vi "ad get drv version.vi"(8 "error in (no error)":errorcluster, 10 "vers":u32, 11 "adh":i32) -> (0 "error out":errorcluster, 2 "vers out":u32, 3 "function return":i32)   [LabVIEW 2021, in "libad4.lvlib"]
doc: "ad_get_drv_version (int32_t adh, uint32_t *vers);\n\nIndicates what version of the DAQ driver LIBAD4 is compatible with."
uses:
  <userlib>/libad4/libad4.lvlib
  <userlib>/libad4/libad4.dll
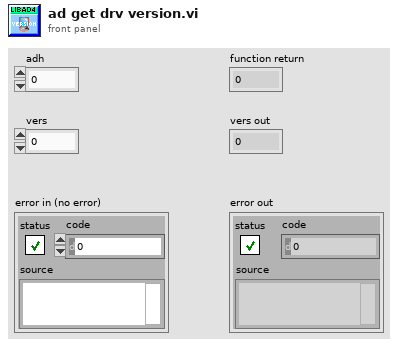
[diagram p1: front panel]
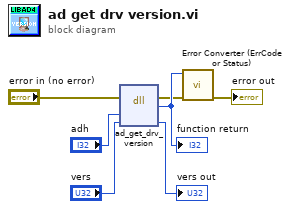
[diagram p0: block diagram]
diagram:
  n1 = dll-call lib="C:/Program Files/National Instruments/LabVIEW 2021/user.lib/libad4/libad4.*" fn="ad_get_drv_version"(error in="error in (no error)", "adh"="adh", "vers"="vers") -> (error out=w2:errorcluster, w7:i32, "vers"=→"vers out":u32)  [unwired: 3 in, 1 out]
  "function return" <- w7
  n2 = call <userlib>:"Error Converter (ErrCode or Status).vi"("error in (no error)"=w2, "error code"=w7) -> ("error out"=→"error out":errorcluster)  [unwired: 9 in]
